vi "UHR-Fleezers Control (host) -Leonardo 04-2018 V1.vi"(0 "Tab Control":T5(tab)=enum."Trap Control (RF)") -> ()   [LabVIEW 2013] (continued)
                }
              }
            }
          }
          frame Enabled {
            n953 = call "hamilton_controller.vi"("Open?"=w1533, "valve"=enum16{"A", "B", "C", "D", "ALL"}."A", "action"=T21."MOVE VALVE") -> ()  [unwired: 8 in, 1 out]
          }
        }
      }
      event "Inject Valve B": Value Change {
        n954 = event-data() -> ()  [unwired: 7 out]
        n955 = disable-structure shown="Enabled" {
          disable-tunnel: "Inject Valve B" -> [w1537 w1557]
          frame Disabled {
            n956 = local read "Pump write delay (ms)"() -> (w1539:dbl)
            n957 = flat-sequence {
              tunnel: w1538 -> [w1552]
              tunnel: w1539 -> [w1548]
              tunnel: w1537 -> [_]
              tunnel: w1539 -> [w1554]
              tunnel: w1538 -> [w1555]
              frame #0 {
                n958 = local read "All Pump Parameters"() -> (w1547:T6)
                n959 = Multiply(x=60.0, y="Flush Center Ch Rate (ul/m)") -> (x*y=w1544:dbl)
                n960 = Unbundle By Name(w1547) -> ("Pump 2"=w1553:T33)
                n961 = call "Set pump parameters.vi"("Pump write delay (ms)"=w1548, "Volume (uL)"="Flush Center Ch Volume (uL)", "Rate (uL/h)"=w1544, "Units"=3.0, "Pump #"=2.0, "Pump Parameters In"=w1553, "VISA resource name"=w1552) -> ("Pump Parameters Out"=w1546:T33)  [unwired: 3 in]
                n962 = Bundle By Name(cluster=w1547, "Pump 2"=w1546) -> (w1545:T6)
                n963 = local write "All Pump Parameters"(w1545) -> ()
                n964 = Add(x="Flush Center Ch Volume (uL)", y="Total Volume\nFlushed (uL)") -> (x+y=w1541:dbl)
                n965 = local write "Total Volume\nFlushed (uL)"(w1541) -> ()
              }
              frame #1 {
                n966 = Wait (ms)(milliseconds to wait=w1554) -> ()  [unwired: 1 out]
              }
              frame #2 {
                n967 = call "Write to pump.vi"("string"="start", "VISA resource name"=w1555) -> ()  [unwired: 1 out]
              }
            }
            n968 = local read "Chemyx Syringe Pump Serial Port"() -> (w1538:refnum<visa-resource-name>)
          }
          frame Enabled {
            n969 = call "hamilton_controller.vi"("Open?"=w1557, "valve"=enum16{"A", "B", "C", "D", "ALL"}."B", "action"=T21."MOVE VALVE") -> ()  [unwired: 8 in, 1 out]
          }
        }
      }
      event "Inject Bottom": Value Change {
        n970 = event-data() -> ()  [unwired: 7 out]
        n971 = call "hamilton_controller.vi"("Open?"="Inject Bottom", "valve"=enum16{"A", "B", "C", "D", "ALL"}."C", "action"=T21."MOVE VALVE") -> ()  [unwired: 8 in, 1 out]
      }
      event "Shunt:": Value Change {
        n972 = event-data() -> ()  [unwired: 7 out]
        n973 = call "hamilton_controller.vi"("Open?"="Shunt:", "valve"=enum16{"A", "B", "C", "D", "ALL"}."D", "action"=T21."MOVE VALVE") -> ()  [unwired: 8 in, 1 out]
      }
      event "Flip Green Filter": Value Change {
        n974 = event-data() -> ()  [unwired: 7 out]
        n975 = local write "Flip Green Filter"("Flip Green Filter") -> ()
        n976 = flat-sequence {
          tunnel: w1573 -> [w1578]
          tunnel: w1572 -> [w1577]
          tunnel: [w1575] -> w1570
          tunnel: [w1574] -> w1569
          tunnel: [w1580] -> w1568
          tunnel: w1570 -> [w1580]
          tunnel: [w1579] -> w1567
          tunnel: w1569 -> [w1579]
          tunnel: w1568 -> [w1584]
          tunnel: w1567 -> [w1583]
          tunnel: [w1582] -> w1571
          frame #0 {
            n977 = xnode "Read/Write Control"("FPGA VI Reference In"=w1578, "error in"=w1577, "Green Filter Flipper"=TRUE) -> ("FPGA VI Reference Out"=w1575:T20, "error out"=w1574:errorcluster)
          }
          frame #1 {
            n978 = Wait (ms)(milliseconds to wait=u32 100) -> ()  [unwired: 1 out]
          }
          frame #2 {
            n979 = xnode "Read/Write Control"("FPGA VI Reference In"=w1584, "error in"=w1583, "Green Filter Flipper"=FALSE) -> ("error out"=w1582:errorcluster)  [unwired: 1 out]
          }
        }
      }
      event "Pump 1 contents", "Pump 3 contents": Value Change {
        n980 = event-data() -> ()  [unwired: 7 out]
        n981 = local read "Pump 1 contents"() -> (→"Pump 1 cont disp":string)
        n982 = local read "Pump 3 contents"() -> (→"Pump 3 cont disp":string)
      }
      event "Reset Trap Pos. FB": Value Change {
        n983 = event-data() -> ()  [unwired: 7 out]
        n984 = xnode "Read/Write Control"("FPGA VI Reference In"=w1590, "error in"=w1589, "Trap Pos. FB Reset"="Reset Trap Pos. FB") -> ()  [unwired: 2 out]
      }
      event "Trap Pos. FB ON": Value Change {
        n985 = event-data() -> ()  [unwired: 7 out]
        n986 = xnode "Read/Write Control"("FPGA VI Reference In"=w1605, "error in"=w1604) -> ("FPGA VI Reference Out"=w1602:T20, "BD1 Frequency Out 1"=w1599:u64)  [unwired: 1 out]
        n987 = To Double Precision Float(number=w1599) -> (double precision float=w1598:dbl)
        n988 = Multiply(x=49125000.0, y=6.0) -> (x*y=w1597:dbl)
        n989 = Multiply(x=w1598, y=w1597) -> (x*y=w1595:dbl)
        n990 = Scale By Power Of 2(n=-48, x=w1595) -> (x*2^n=w1594:dbl)
        n991 = Divide(x=w1594, y=1000000.0) -> (x/y=w1591:dbl)
        n992 = flat-sequence {
          tunnel: [w1608] -> w1603
          tunnel: w1602 -> [w1609]
          tunnel: w1599 -> [w1607]
          tunnel: "Trap Pos. FB ON" -> [w1606]
          tunnel: "Trap Pos. FB ON" -> [w1615]
          tunnel: w1603 -> [w1614]
          tunnel: "Trap Pos. FB ON" -> [w1617]
          tunnel: w1591 -> [w1616]
          frame #0 {
            n993 = case shown="False" w1606 {
              tunnel: w1609 -> [w1612 w1613]
              tunnel: [w1611 w1613] -> w1608
              tunnel: w1607 -> [w1610 _]
              frame False {
                n994 = xnode "Read/Write Control"("FPGA VI Reference In"=w1612, "BD 1 Frequency 1"=w1610) -> ("FPGA VI Reference Out"=w1611:T20)  [unwired: 1 in, 1 out]
              }
              frame True {
              }
            }
          }
          frame #1 {
            n995 = xnode "Read/Write Control"("FPGA VI Reference In"=w1614, "Force feedback"=w1615) -> ()  [unwired: 1 in, 2 out]
          }
          frame #2 {
            n996 = case shown="False" w1617 {
              tunnel: w1616 -> [w1620 _]
              frame False {
                n997 = local read "T2 for asymmetric\n(MHz)"() -> (w1618:dbl)
                n998 = Subtract(x=w1618, y=w1620) -> (x-y=w1619:dbl)
                n999 = property on="Trap Delta (MHz)" class="DigNum (strict)"("Val(Sgnl)"=w1619) -> ()  [unwired: 2 in, 2 out]
              }
              frame True {
              }
            }
          }
        }
      }
      event "Diff. FB.", "Trap Pos. FB Gains", "Trap Pos. FB Mult Factor", "Trap Pos. FB Offset Factor", "Trap Pos FB Negate Action", "Trap Pos FB Monitor\nT1 or T2", "Negate Diff?": Value Change {
        n1000 = event-data() -> ()  [unwired: 7 out]
        n1001 = xnode "Read/Write Control"("FPGA VI Reference In"=w1631, "error in"=w1630, "Trap pos. FB Range"="Trap Pos. FB Range", "Trap Pos. FB Gains"="Trap Pos. FB Gains", "Trap Pos. FB Mult Factor"="Trap Pos. FB Mult Factor", "Trap Pos. FB Offset Factor"="Trap Pos. FB Offset Factor", "Trap Pos FB Negate Action"="Trap Pos FB Negate Action", "Trap Pos FB Monitor T1 or T2"="Trap Pos FB Monitor\nT1 or T2", "AI1 X Scale"="Trap Pos. AI1 X Pre-scale", "Negate Diff?"="Negate Diff?", "Diff FB Measurement?"="Diff. FB.") -> ()  [unwired: 2 out]
      }
      event "Trap Pos FB SP": Value Change {
        n1002 = event-data() -> ()  [unwired: 7 out]
        n1003 = xnode "Read/Write Control"("FPGA VI Reference In"=w1634, "error in"=w1633, "Trap Pos. FB SP"="Trap Pos FB SP") -> ()  [unwired: 2 out]
        n1004 = disable-structure shown="Disabled" {
          frame Disabled {
            n1005 = local read "Trap X AI1 (DMA)"() -> (w1655:T13)
            n1006 = local read "Trap X (AI1)"() -> (w1656:T1)
            n1007 = local read "Setpoint offset\nCorrection values"() -> (w1649:dbl[])
            n1008 = local read "Trap Delta (MHz)"() -> (w1653:dbl)
            n1009 = local read "B factor"() -> (w1640:dbl)
            n1010 = Unbundle(w1656) -> ("Trap 1"=w1654:fxp<+/-,16,1>, "Trap 2"=w1643:fxp<+/-,16,1>)
            n1011 = Unbundle(w1655) -> ("Set 1"=w1639:fxp<+/-,16,1>, "Set 2"=w1638:fxp<+/-,16,1>)
            n1012 = Negate(x=w1643) -> (-x=w1636:fxp<+/-,17,2>)
            n1013 = Negate(x=w1654) -> (-x=w1637:fxp<+/-,17,2>)
            n1014 = Divide(x=w1653, y=0.1) -> (x/y=w1651:dbl)
            n1015 = Multiply(x=w1638, y=w1640) -> (x*y=w1641:dbl)
            n1016 = Subtract(x=w1639, y=w1641) -> (x-y=w1646:dbl)
            n1017 = To Long Integer(number=w1651) -> (32bit integer=w1650:i32)
            n1018 = Index Array(array=w1649, index=w1650) -> (element=w1645:dbl)
            n1019 = Multiply(x=w1640, y=w1636) -> (x*y=w1642:dbl)
            n1020 = Subtract(x=w1637, y=w1642) -> (x-y=w1648:dbl)
            n1021 = Add(x=w1648, y=w1645) -> (x+y=→"ideal setpoint fpga":dbl)
            n1022 = Add(x=w1646, y=w1645) -> (x+y=→"ideal setpoint avgd":dbl)
          }
          frame Enabled {
          }
        }
        n1023 = disable-structure shown="Enabled" {
          frame Enabled {
          }
          frame Disabled {
            n1024 = local write "B factor"(1.0 ("B factor")) -> ()
          }
        }
      }
      event "Simulate stepping": Value Change {
        n1025 = event-data() -> ()  [unwired: 7 out]
        n1026 = flat-sequence {
          tunnel: w1658 -> [w1661]
          tunnel: [w1660] -> _
          tunnel: w1657 -> [w1659]
          frame #0 {
            n1027 = while {
              tunnel: w1661 -> [w1689]
              tunnel: [w1688] -> w1660 mode=indexing
              tunnel: w1659 -> [w1687]
              i -> [w1673]
              stop <- w1670 stop-if-true
              w1663 = 1000.0
              n1028 = Divide(x="Backtrack probability", y=100) -> (x/y=w1697:dbl)
              n1029 = Random Number (0-1)() -> (number: 0 to 1=w1698:dbl)
              n1030 = Greater?(x=w1698, y=w1697) -> (0:w1696:bool)
              n1031 = Select(t=1, s=w1696, f=-1) -> (s? t:f=w1693:i32)
              n1032 = local read "BD 1 Frequency 2 (MHz)"() -> (w1668:dbl)
              n1033 = Multiply(x=w1693, y="Step size (nm)") -> (x*y=w1691:dbl)
              "Step taken" <- w1691
              n1034 = Divide(x=w1691, y=168.33) -> (x/y=w1666:dbl)
              n1035 = local read "BD 1 Frequency 1 (MHz)"() -> (w1667:dbl)
              n1036 = local read "X RF Frequency Limits (MHz)"() -> (w1686:T16)
              n1037 = local read "Y RF Frequency Limits (MHz)"() -> (w1685:T16)
              n1038 = Subtract(x=w1667, y=w1666) -> (x-y=w1665:dbl)
              n1039 = local write "BD 1 Frequency 1 (MHz)"(w1665) -> ()
              n1040 = local read "BD 2 Frequency 1 (MHz)"() -> (w1683:dbl)
              n1041 = local read "BD 2 Frequency 2 (MHz)"() -> (w1684:dbl)
              n1042 = call "set RF board frequency - interlace.vi"("Board 2 Frequency Limits"=w1685, "Board 1 Frequency Limits"=w1686, "error in"=w1689, "FPGA VI Reference In"=w1687, "Board 2 Frequency 2 (MHz)"=w1684, "Board 2 Frequency 1 (MHz)"=w1683, "Board 1 Frequency 2 (MHz)"=w1668, "Board 1 Frequency 1  (MHz)"=w1665) -> ("error out"=w1688:errorcluster)  [unwired: 2 in, 1 out]
              n1043 = Subtract(x=w1668, y=w1665) -> (x-y=w1682:dbl)
              n1044 = Subtract(x=w1684, y=w1683) -> (x-y=w1681:dbl)
              n1045 = Square(x=w1681) -> (x^2=w1679:dbl)
              n1046 = Square(x=w1682) -> (x^2=w1680:dbl)
              n1047 = Add(x=w1680, y=w1679) -> (x+y=w1678:dbl)
              n1048 = Square Root(x=w1678) -> (sqrt(x)=w1669:dbl)
              n1049 = local write "Trap Delta (MHz)"(w1669) -> ()
              n1050 = property on="Initial delta (MHz)" class="DigNum (strict)"("Val(Sgnl)"=w1669) -> ()  [unwired: 2 in, 2 out]
              n1051 = Multiply(x="Mean dwell time (s)", y=w1663) -> (x*y=w1675:dbl)
              n1052 = case shown="\"Gamma2\"" "Distribution" {
                tunnel: w1675 -> [w1702 w1706 w1709]
                tunnel: [w1702 w1703 w1710] -> w1664
                frame "uniform", Default {
                }
                frame "Exponential" {
                  n1053 = call-poly <vilib>:"Continuous Random.vi"("b"=w1706, "samples"=1) -> ("exp random data"=w1704:dbl[])  [unwired: 8 in, 1 out]
                  n1054 = Index Array(array=w1704) -> (element=w1703:dbl)  [unwired: 1 in]
                }
                frame "Gamma2" {
                  w1707 = 2.0
                  # "Note: the shape and scale\nparameters of the gamma\nare inverted because LabView..."
                  n1055 = Divide(x=w1709, y=w1707) -> (x/y=w1708:dbl)
                  n1056 = call-poly <vilib>:"Continuous Random.vi"("c"=w1708, "b"=w1707, "samples"=1) -> ("gamma random numbers"=w1711:dbl[])  [unwired: 7 in, 1 out]
                  n1057 = Index Array(array=w1711) -> (element=w1710:dbl)  [unwired: 1 in]
                }
              }
              n1058 = Divide(x=w1664, y=w1663) -> (x/y=→"Step duration":dbl)
              n1059 = To Unsigned Long Integer(number=w1664) -> (unsigned 32bit integer=w1676:u32)
              n1060 = Add(x=w1673, y=1) -> (x+y=w1672:i32)
              n1061 = Wait (ms)(milliseconds to wait=w1676) -> ()  [unwired: 1 out]
              n1062 = Equal?(x=w1672, y="Number of steps") -> (x = y?=w1670:bool)
            }
          }
          frame #1 {
            n1063 = local write "Simulate stepping"(FALSE) -> ()
          }
        }
      }
      event "Set SP to Reading": Value Change {
        n1064 = event-data() -> ()  [unwired: 7 out]
        n1065 = local read "Trap Pos FB Monitor\nT1 or T2"() -> (w1721:bool)
        n1066 = local read "Trap X AI1 (DMA)"() -> (w1724:T13)
        n1067 = local read "Trap X (AI1)"() -> (w1727:T1)
        n1068 = Unbundle By Name(w1727) -> ("Trap 1"=w1726:fxp<+/-,16,1>, "Trap 2"=w1725:fxp<+/-,16,1>)
        n1069 = Unbundle By Name(w1724) -> ("Set 1"=w1723:fxp<+/-,16,1>, "Set 2"=w1722:fxp<+/-,16,1>)
        n1070 = Select(t=w1726, s=w1721, f=w1725) -> (s? t:f=w1720:fxp<+/-,16,1>)
        n1071 = Select(t=w1723, s=w1721, f=w1722) -> (s? t:f=w1719:fxp<+/-,16,1>)
        n1072 = Not(x="Set SP Using...") -> (.not. x?=w1714:bool)
        n1073 = Select(t=w1720, s=w1714, f=w1719) -> (s? t:f=w1715:fxp<+/-,16,1>)
        n1074 = xnode "Read/Write Control"("FPGA VI Reference In"=w1717, "error in"=w1716, "Trap Pos. FB SP"=w1715) -> ()  [unwired: 2 out]
        n1075 = local write "Trap Pos FB SP"(w1715) -> ()
      }
      event "Trap Pos. FB Out Scale 2^n": Value Change {
        n1076 = event-data() -> ()  [unwired: 7 out]
        n1077 = Scale By Power Of 2(n="Trap Pos. FB Out Scale 2^n", x=ext 1.0) -> (x*2^n=w1729:ext)
        n1078 = property on="Trap Pos. FB Mult Factor" class="DigNum (strict)"("Val(Sgnl)"=w1729) -> ()  [unwired: 2 in, 2 out]
      }
      event "Trap Pos FB Int Count": Value Change {
        n1079 = event-data() -> ()  [unwired: 7 out]
        n1080 = xnode "Read/Write Control"("FPGA VI Reference In"=w1734, "error in"=w1733, "Trap Pos FB Int Count"="Trap Pos FB Int Count") -> ()  [unwired: 2 out]
      }
      event "Target Force (pN)", "Setpoint offset\nCorrection values", "Raster target force (pN)": Value Change {
        w1743 = 2.0
        n1081 = event-data() -> ()  [unwired: 7 out]
        n1082 = disable-structure "Removed B Factor to improve position feedback - Alex 081418 1of3" shown="Enabled" {
          disable-tunnel: [w1773 fxp<+/-,32,16> 1.0 ("B factor")] -> w1735
          frame Disabled {
            n1083 = local read "B factor"() -> (w1774:dbl)
            n1084 = To Fixed-Point(number=w1774) -> (fixed-point=w1773:fxp<+/-,16,16>)  [unwired: 1 in]
          }
          frame Enabled {
          }
        }
        n1085 = xnode "Read/Write Control"("FPGA VI Reference In"=w1737, "B factor"=w1735) -> ("BD1 Frequency Out 1"=w1764:u64)  [unwired: 1 in, 2 out]
        n1086 = local read "BD 1 Frequency 2 (MHz)"() -> (w1763:dbl)
        n1087 = local read "Target Force (pN)"() -> (w1749:dbl)
        n1088 = To Double Precision Float(number=w1764) -> (double precision float=w1770:dbl)
        n1089 = Multiply(x=49125000.0, y=6.0) -> (x*y=w1769:dbl)
        n1090 = Multiply(x=w1770, y=w1769) -> (x*y=w1767:dbl)
        n1091 = Scale By Power Of 2(n=-48, x=w1767) -> (x*2^n=w1766:dbl)
        n1092 = Divide(x=w1766, y=1000000.0) -> (x/y=w1762:dbl)
        n1093 = Subtract(x=w1763, y=w1762) -> (x-y=w1761:dbl)
        n1094 = local read "T1 kappa_x (pN/nm)"() -> (w1750:dbl)
        n1095 = local read "T1 alpha_x (nm/V)"() -> (w1751:dbl)
        n1096 = local read "Negate offset difference"() -> (w1752:bool)
        n1097 = local read "Offset file step size"() -> (w1760:dbl)
        n1098 = Multiply(x="Raster target force (pN)", y=w1743) -> (x*y=w1742:dbl)
        n1099 = Multiply(x=w1749, y=w1743) -> (x*y=w1748:dbl)
        n1100 = local read "Setpoint offset\nCorrection values"() -> (w1757:dbl[])
        n1101 = Divide(x=w1761, y=w1760) -> (x/y=w1759:dbl)
        n1102 = Select(t=-1, s=w1752, f=1) -> (s? t:f=w1753:i32)
        n1103 = To Long Integer(number=w1759) -> (32bit integer=w1758:i32)
        n1104 = Multiply(x=w1751, y=w1750) -> (x*y=w1741:dbl)
        n1105 = Divide(x=w1748, y=w1741) -> (x/y=w1747:dbl)
        n1106 = Index Array(array=w1757, index=w1758) -> (element=w1756:dbl)
        n1107 = Divide(x=w1742, y=w1741) -> (x/y=w1740:dbl)
        n1108 = Multiply(x=w1753, y=w1756) -> (x*y=w1739:dbl)
        n1109 = Add(x=w1747, y=w1739) -> (x+y=w1746:dbl)
        n1110 = Add(x=w1740, y=w1739) -> (x+y=w1738:dbl)
        n1111 = To Fixed-Point(number=w1738) -> (fixed-point=w1736:fxp<+/-,16,1>)  [unwired: 1 in]
        n1112 = To Fixed-Point(number=w1746) -> (fixed-point=w1745:fxp<+/-,16,1>)  [unwired: 1 in]
        n1113 = property on="Trap Pos FB SP" class="DigNum (strict)"("Val(Sgnl)"=w1745) -> ()  [unwired: 2 in, 2 out]
        n1114 = xnode "Read/Write Control"("FPGA VI Reference In"=w1737, "Raster setpoint"=w1736) -> ()  [unwired: 1 in, 2 out]
      }
      event "Read setpoint correction\nfile": Value Change {
        n1115 = event-data() -> ()  [unwired: 7 out]
        n1116 = local write "Read setpoint correction\nfile"(FALSE) -> ()
        n1117 = Open/Create/Replace File(file path (use dialog)="Setpoint correction\noffset file", operation (0:open)=T24."open", access (0:read/write)=enum16{"read/write", "read-only", "write-only"}."read-only") -> (refnum out=w1801:refnum<file>)  [unwired: 1 in, 4 out]
        n1118 = Deny Access(7:w1801) -> (3:w1799:refnum<file>)  [unwired: 1 in, 2 out]
        n1119 = Read from Binary File(5:0.0, 9:T30."big-endian, network order" ("byte order (0:big-endian, network order)"), 10:-1 ("count (1)"), 11:w1799) -> (2:w1792:dbl[], 3:w1798:refnum<file>)  [unwired: 1 in, 3 out]
        n1120 = Close File(refnum=w1798) -> ()  [unwired: 1 in, 2 out]
        n1121 = Index Array(array=w1792, index=0) -> (element=w1788:dbl)
        n1122 = local write "Offset file step size"(w1788) -> ()
        n1123 = Array Subset(array=w1792, index=3) -> (w1791:dbl[])  [unwired: 1 in]
        n1124 = local read "T1 kappa_x (pN/nm)"() -> (w1786:dbl)
        n1125 = local read "T1 alpha_x (nm/V)"() -> (w1787:dbl)
        n1126 = local read "T2 alpha_x (nm/V)"() -> (w1785:dbl)
        n1127 = local read "T2 kappa_x (pN/nm)"() -> (w1784:dbl)
        n1128 = Decimate 1D Array(w1791) -> (w1780:dbl[], w1781:dbl[])  [unwired: 1 out]
        n1129 = local read "Offset Values"() -> (w1790:T14)
        n1130 = Multiply(x=w1787, y=w1786) -> (x*y=w1782:dbl)
        n1131 = Multiply(x=w1785, y=w1784) -> (x*y=w1783:dbl)
        n1132 = Bundle By Name(cluster=w1790, "Trap 1X offset"=w1780, "Trap 2X offset"=w1781) -> (w1789:T14)
        n1133 = Divide(x=w1783, y=w1782) -> (x/y=w1777:dbl)
        n1134 = disable-structure "Removed B Factor to better position FB - Alex 081418 3of3" shown="Enabled" {
          disable-tunnel: w1777 -> [w1805 _]
          disable-tunnel: [w1805 1.0] -> w1776
          frame Disabled {
          }
          frame Enabled {
          }
        }
        n1135 = Multiply(x=w1781, y=w1776) -> (x*y=w1779:dbl[])
        n1136 = local write "Offset Values"(w1789) -> ()
        n1137 = Subtract(x=w1780, y=w1779) -> (x-y=w1778:dbl[])
        n1138 = property on="B factor" class="DigNum (strict)"("Val(Sgnl)"=w1776) -> ()  [unwired: 2 in, 2 out]
        n1139 = property on="Setpoint offset\nCorrection values" class="Arr (strict)"("Val(Sgnl)"=w1778) -> ()  [unwired: 2 in, 2 out]
      }
      event "MCL Tracking": Value Change {
        n1140 = event-data() -> ()  [unwired: 7 out]
        n1141 = case shown="True" "MCL Tracking" {
          frame False {
            n1142 = local read "Current MCL (V)"() -> (w1808:dbl)
            n1143 = local write "AO2"(w1808) -> ()
          }
          frame True {
            n1144 = local read "BD 1 Frequency 1 (MHz)"() -> (→"Zero T1 position":dbl)
            n1145 = local read "AO2"() -> (→"Zero MCL x position":dbl)
          }
        }
      }
      event "Scale intensities": Value Change {
        n1146 = event-data() -> ()  [unwired: 7 out]
        n1147 = local read "Trap Intensity\nSetpoints (V)"() -> (w1814:cluster{"Set 1":dbl, "Set 2":dbl})
        n1148 = local read "T1 kappa_x (pN/nm)"() -> (w1820:dbl)
        n1149 = local read "T2 kappa_x (pN/nm)"() -> (w1819:dbl)
        n1150 = Unbundle By Name(w1814) -> ("Set 1"=w1816:dbl, "Set 2"=w1815:dbl)
        n1151 = case shown="True" "Scale intensities" {
          tunnel: "Scale factor" -> [w1830 w1842]
          tunnel: "Scale factor" -> [w1825 w1835]
          tunnel: w1820 -> [w1832 w1841]
          tunnel: w1819 -> [w1831 w1840]
          tunnel: [w1828 w1839] -> w1818
          tunnel: [w1829 w1838] -> w1817
          tunnel: w1816 -> [w1827 w1837]
          tunnel: w1815 -> [w1826 w1836]
          tunnel: [w1824 w1834] -> w1813
          tunnel: [w1823 w1833] -> w1812
          frame False {
            n1152 = Divide(x=w1832, y=w1825) -> (x/y=w1828:dbl)
            n1153 = Divide(x=w1831, y=w1830) -> (x/y=w1829:dbl)
            n1154 = Divide(x=w1827, y=w1825) -> (x/y=w1824:dbl)
            n1155 = Divide(x=w1826, y=w1825) -> (x/y=w1823:dbl)
          }
          frame True {
            n1156 = Multiply(x=w1837, y=w1835) -> (x*y=w1834:dbl)
            n1157 = Multiply(x=w1836, y=w1835) -> (x*y=w1833:dbl)
            n1158 = Multiply(x=w1841, y=w1835) -> (x*y=w1839:dbl)
            n1159 = Multiply(x=w1842, y=w1840) -> (x*y=w1838:dbl)
          }
        }
        n1160 = local write "T2 kappa_x (pN/nm)"(w1817) -> ()
        n1161 = local write "T1 kappa_x (pN/nm)"(w1818) -> ()
        n1162 = Bundle By Name(cluster=w1814, "Set 1"=w1813, "Set 2"=w1812) -> (w1811:cluster{"Set 1":dbl, "Set 2":dbl})
        n1163 = property on="Trap Intensity\nSetpoints (V)" class="Clust (strict)"("Val(Sgnl)"=w1811) -> ()  [unwired: 2 in, 2 out]
      }
    }
    "error out 2" <- w771
    n1164 = node-c288() -> ()  [unwired: 1 in, 1 out]
  }
  n1165 = node-c288() -> (w102:T25)  [unwired: 4 in]
  n1166 = timed-loop "Run Scripts, including: stage motion" {
    timing: w102 -> [_]
    timing-out: [_] -> w101
    tunnel: w59 -> [_]
    stop <- w1844 stop-if-true
    n1167 = node-c288() -> ()  [unwired: 1 in, 1 out]
    n1168 = event shown="[2] \"Cal/Data Acq. Spot\": Value Change" {
      selector: _ -> [_ _ _ _ _ _ _ _ _ _ _ _]
      dyn-events: _ -> [_ _ _ _ _ _ _ _ _ _ _ _]
      timeout: 50 -> [_ _ _ _ _ _ _ _ _ _ _ _]
      tunnel: ["Move Cap. 1 (DNA Top)" _ "Cal/Data Acq. Spot" "Dump Beads" "Dip for Protein" _ "Got ADig bead" "Got DNA bead" "Take Stepping Data" _ "Take Detection Laser\nImage" _] -> _
      tunnel: [_ _ _ _ _ _ _ _ _ _ _ w2054] -> w1844
      event "Move Cap. 1 (DNA Top)": Value Change {
        n1169 = event-data() -> ()  [unwired: 1 in, 5 out]
        n1170 = local write "Move Cap. 1 (DNA Top)"(FALSE ("Move Cap. 1 (DNA Right)")) -> ()
        n1171 = flat-sequence {
          tunnel: "Cap 1 Samp Flow ON" -> [w1850]
          frame #0 {
            n1172 = local write "Stage Moving"(FALSE ("Stage Moving")) -> ()
            n1173 = case "stop flow" shown="True" w1850 {
              frame False {
              }
              frame True {
                n1174 = call "hamilton_controller.vi"("Open?"=FALSE, "valve"=enum16{"A", "B", "C", "D", "ALL"}."C", "action"=T21."MOVE VALVE") -> ()  [unwired: 8 in, 1 out]
              }
            }
            n1175 = case shown="True" TRUE {
              tunnel: "Cap 1 T ON" -> [w1859 w1860]
              frame False {
                n1176 = property on="Trap 1 (ON/OFF)" class="Bool (strict)"("Val(Sgnl)"=w1859) -> ()  [unwired: 2 in, 2 out]
              }
              frame True {
                n1177 = property on="Trap 2 (ON/OFF)" class="Bool (strict)"("Val(Sgnl)"=w1860) -> ()  [unwired: 2 in, 2 out]
              }
            }
            n1178 = call <vilib>:"Beep.vi"() -> ()  [unwired: 3 in, 9 out]
            n1179 = case shown="True" "Cap 1 Flow ON" {
              frame False {
              }
              frame True {
                n1180 = property on="Main:" class="Bool (strict)"("Val(Sgnl)"=TRUE ("Value (Signaling)")) -> ()  [unwired: 2 in, 2 out]
              }
            }
          }
        }
      }
      event Timeout {
        n1181 = event-data() -> ()  [unwired: 1 in, 2 out]
      }
      event "Cal/Data Acq. Spot": Value Change {
        # "wait for calibration file\nto be written"
        # "signal save cal true\nthis tells the data \nacquisition loop to\nstart sending the data\nto a calibration file"
        # "separate traps to\nthe desired trap delta"
        # "move stage to data acquisition spot"
        # "CHANGE FISH FOR TETHER BACK\nTO TRUE VALUE HERE."
        n1182 = event-data() -> ()  [unwired: 1 in, 5 out]
        n1183 = flat-sequence {
          tunnel: ["Cal @ (MHz)"] -> w1861
          tunnel: w1861 -> [w1873]
          tunnel: w1861 -> [w1894]
          frame #0 {
            n1184 = property on="Trap Delta (MHz)" class="DigNum (strict)"("Val(Sgnl)"="Cal @ (MHz)") -> ()  [unwired: 2 in, 2 out]
            n1185 = call <vilib>:"Beep.vi"() -> ()  [unwired: 3 in, 9 out]
          }
          frame #1 {
            n1186 = local read "Scale intensities"() -> (w1865:bool)
            n1187 = case shown="True" w1865 {
              frame False {
              }
              frame True {
                n1188 = property on="Scale intensities" class="Bool (strict)"("Val(Sgnl)"=FALSE ("Value (Signaling)")) -> ()  [unwired: 2 in, 2 out]
              }
            }
            n1189 = Wait (ms)(milliseconds to wait=u32 250) -> ()  [unwired: 1 out]
          }
          frame #2 {
            n1190 = property on="Save Calibration" class="Bool (strict)"("Val(Sgnl)"=TRUE ("Value (Signaling)")) -> ()  [unwired: 2 in, 2 out]
          }
          frame #3 {
            n1191 = Wait (ms)(milliseconds to wait=u32 4000) -> ()  [unwired: 1 out]
          }
          frame #4 {
            n1192 = while {
              stop <- w1870 stop-if-true
              n1193 = local read "Saving..."() -> (w1871:bool)
              n1194 = Wait (ms)(milliseconds to wait=u32 100) -> ()  [unwired: 1 out]
              n1195 = Not(x=w1871) -> (.not. x?=w1870:bool)
            }
          }
          frame #5 {
            n1196 = case shown="True" "W/ Offset 1" {
              tunnel: w1873 -> [_ w1875]
              frame False {
              }
              frame True {
                n1197 = stacked-sequence {
                  tunnel: w1875 -> [_ _ _ _ _ _ _ w1892]
                  frame #0 {
                    n1198 = Replace Array Subset(array=u32[] [0] ("Index Values"), new element="Offset 1 Set", index=0) -> (w1876:u32[])
                    n1199 = property on="Saved AOD Raster Scan Parameter Sets" class="Arr (strict)"("Index Values"=w1876) -> ()  [unwired: 2 in, 2 out]
                    n1200 = property on="Trap Delta (MHz)" class="DigNum (strict)"("Val(Sgnl)"="Offset 1 Start (MHz)") -> ()  [unwired: 2 in, 2 out]
                  }
                  frame #1 {
                    n1201 = Wait (ms)(milliseconds to wait=u32 200) -> ()  [unwired: 1 out]
                  }
                  frame #2 {
                    n1202 = property on="Load parameters" class="Bool (strict)"("Val(Sgnl)"=TRUE ("Value (Signaling)")) -> ()  [unwired: 2 in, 2 out]
                  }
                  frame #3 {
                    n1203 = Wait (ms)(milliseconds to wait=u32 200) -> ()  [unwired: 1 out]
                  }
                  frame #4 {
                    n1204 = property on="Trap Raster Scan" class="Bool (strict)"("Val(Sgnl)"=TRUE ("Value (Signaling)")) -> ()  [unwired: 2 in, 2 out]
                  }
                  frame #5 {
                    n1205 = Wait (ms)(milliseconds to wait=u32 2000) -> ()  [unwired: 1 out]
                  }
                  frame #6 {
                    n1206 = while {
                      stop <- w1889 stop-if-true
                      n1207 = local read "Raster Scanning..."() -> (w1891:bool)
                      n1208 = local read "Saving..."() -> (w1887:bool)
                      n1209 = Wait (ms)(milliseconds to wait=u32 100) -> ()  [unwired: 1 out]
                      n1210 = Not(x=w1887) -> (.not. x?=w1886:bool)
                      n1211 = Not(x=w1891) -> (.not. x?=w1888:bool)
                      n1212 = And(x=w1888, y=w1886) -> (x .and. y?=w1889:bool)
                    }
                  }
                  frame #7 {
                    n1213 = property on="Trap Delta (MHz)" class="DigNum (strict)"("Val(Sgnl)"=w1892) -> ()  [unwired: 2 in, 2 out]
                  }
                }
              }
            }
          }
          frame #6 {
            n1214 = local read "Save ave N"() -> (w1893:dbl)
            n1215 = case shown="True" "W/ Offset 2" {
              tunnel: w1894 -> [_ w1900]
              tunnel: w1893 -> [_ w1899]
              frame False {
                n1216 = Multiply(x="Cal read wait (s)", y=u32 1000 ("milliseconds to wait")) -> (x*y=w1897:u32)
                n1217 = Wait (ms)(milliseconds to wait=w1897) -> ()  [unwired: 1 out]
              }
              frame True {
                n1218 = stacked-sequence {
                  tunnel: w1900 -> [_ _ _ _ _ _ _ _ _ w1921 _ _]
                  tunnel: w1899 -> [_ _ _ _ _ _ _ _ _ w1919 _ _]
                  frame #0 {
                    n1219 = property on="Save ave N" class="DigNum (strict)"("Val(Sgnl)"=1.0 ("Value (Signaling)")) -> ()  [unwired: 2 in, 2 out]
                  }
                  frame #1 {
                    n1220 = Wait (ms)(milliseconds to wait=u32 500) -> ()  [unwired: 1 out]
                  }
                  frame #2 {
                    n1221 = property on="Trap Delta (MHz)" class="DigNum (strict)"("Val(Sgnl)"="Offset 2 Start (MHz)") -> ()  [unwired: 2 in, 2 out]
                    n1222 = Replace Array Subset(array=u32[] [0] ("Index Values"), new element="Offset 2 Set", index=0) -> (w1905:u32[])
                    n1223 = property on="Saved AOD Raster Scan Parameter Sets" class="Arr (strict)"("Index Values"=w1905) -> ()  [unwired: 2 in, 2 out]
                  }
                  frame #3 {
                    n1224 = Wait (ms)(milliseconds to wait=u32 500) -> ()  [unwired: 1 out]
                  }
                  frame #4 {
                    n1225 = property on="Load parameters" class="Bool (strict)"("Val(Sgnl)"=TRUE ("Value (Signaling)")) -> ()  [unwired: 2 in, 2 out]
                  }
                  frame #5 {
                    n1226 = Wait (ms)(milliseconds to wait=u32 500) -> ()  [unwired: 1 out]
                  }
                  frame #6 {
                    n1227 = property on="Trap Raster Scan" class="Bool (strict)"("Val(Sgnl)"=TRUE ("Value (Signaling)")) -> ()  [unwired: 2 in, 2 out]
                  }
                  frame #7 {
                    n1228 = Wait (ms)(milliseconds to wait=u32 2000) -> ()  [unwired: 1 out]
                  }
                  frame #8 {
                    n1229 = while {
                      stop <- w1914 stop-if-true
                      n1230 = local read "Raster Scanning..."() -> (w1917:bool)
                      n1231 = local read "Saving..."() -> (w1915:bool)
                      n1232 = Wait (ms)(milliseconds to wait=u32 100) -> ()  [unwired: 1 out]
                      n1233 = Not(x=w1915) -> (.not. x?=w1913:bool)
                      n1234 = Not(x=w1917) -> (.not. x?=w1916:bool)
                      n1235 = And(x=w1916, y=w1913) -> (x .and. y?=w1914:bool)
                    }
                  }
                  frame #9 {
                    n1236 = property on="Trap Delta (MHz)" class="DigNum (strict)"("Val(Sgnl)"=w1921) -> ()  [unwired: 2 in, 2 out]
                    n1237 = property on="Saved AOD Raster Scan Parameter Sets" class="Arr (strict)"("Index Values"=u32[] [0]) -> ()  [unwired: 2 in, 2 out]
                    n1238 = property on="Save ave N" class="DigNum (strict)"("Val(Sgnl)"=w1919) -> ()  [unwired: 2 in, 2 out]
                  }
                  frame #10 {
                    n1239 = Wait (ms)(milliseconds to wait=u32 500) -> ()  [unwired: 1 out]
                  }
                  frame #11 {
                    n1240 = property on="Load parameters" class="Bool (strict)"("Val(Sgnl)"=TRUE ("Value (Signaling)")) -> ()  [unwired: 2 in, 2 out]
                  }
                }
              }
            }
          }
          frame #7 {
            n1241 = property on="Read Cal" class="Bool (strict)"("Val(Sgnl)"=TRUE ("Value (Signaling)")) -> ()  [unwired: 2 in, 2 out]
          }
          frame #8 {
            n1242 = Wait (ms)(milliseconds to wait=u32 500) -> ()  [unwired: 1 out]
          }
          frame #9 {
            n1243 = property on="Fish for Tether" class="Bool (strict)"("Val(Sgnl)"=FALSE ("Value (Signaling)")) -> ()  [unwired: 2 in, 2 out]
          }
        }
        n1244 = local write "Cal/Data Acq. Spot"(FALSE ("Cal/Data Acq. Spot")) -> ()
      }
      event "Dump Beads": Value Change {
        # "SCRIPT TO REMOVE BOTH BEADS FROM THE TRAPS. TURNS ON LIGHT WHICH INDICATES THAT STAGE IS MOVING. THEN STOPS SAVING DATA. \nSETS Sample Channel Flow TO TRUE. STOPS INTERLACING GREEN FLUORESCENCE. TURNS OFF Tether INDICATOR BECAUSE WE ARE THROWING IT\nAWAY. SHUTS OFF TRAP POSITION FEEDBACK."
        n1245 = event-data() -> ()  [unwired: 1 in, 5 out]
        n1246 = flat-sequence {
          frame #0 {
            w1928 = FALSE ("Fl. Triggered...")
            w1929 = TRUE ("Stage Moving")
            n1247 = local read "Saving..."() -> (w1930:bool)
            n1248 = local write "Fl. Triggered..."(w1928) -> ()
            n1249 = local write "Stage Moving"(w1929) -> ()
            n1250 = local write "Tether"(w1928) -> ()
            n1251 = property on="Green Laser ON/Interlacing" class="Bool (strict)"("Val(Sgnl)"=w1928) -> ()  [unwired: 2 in, 2 out]
            n1252 = property on="Trap Pos. FB ON" class="Bool (strict)"("Val(Sgnl)"=w1928) -> ()  [unwired: 2 in, 2 out]
            n1253 = property on="Inject Bottom" class="Bool (strict)"("Val(Sgnl)"=w1929) -> ()  [unwired: 2 in, 2 out]
            n1254 = local write "Stop Saving"(w1930) -> ()
          }
          frame #1 {
            w1931 = FALSE ("Value (Signaling)")
            # "TURNS TRAPS OFF SO THAT\nBEADS REMAIN AT DUMP \nBEADS POSITION"
            n1255 = property on="Trap 1 (ON/OFF)" class="Bool (strict)"("Val(Sgnl)"=w1931) -> ()  [unwired: 2 in, 2 out]
            n1256 = property on="Trap 2 (ON/OFF)" class="Bool (strict)"("Val(Sgnl)"=w1931) -> ()  [unwired: 2 in, 2 out]
            n1257 = call <vilib>:"Beep.vi"() -> ()  [unwired: 3 in, 9 out]
          }
          frame #2 {
            n1258 = property on="Goto Bottom (F7)" class="Bool (strict)"("Val(Sgnl)"=TRUE ("Value (Signaling)")) -> ()  [unwired: 2 in, 2 out]
          }
          frame #3 {
            n1259 = Wait (ms)(milliseconds to wait=u32 8000) -> ()  [unwired: 1 out]
          }
          frame #4 {
            n1260 = property on="Trap Delta (MHz)" class="DigNum (strict)"("Val(Sgnl)"=20.0 ("Value (Signaling)")) -> ()  [unwired: 2 in, 2 out]
          }
          frame #5 {
            n1261 = property on="Trap 2 (ON/OFF)" class="Bool (strict)"("Val(Sgnl)"=TRUE ("Value (Signaling)")) -> ()  [unwired: 2 in, 2 out]
          }
          frame #6 {
            n1262 = property on="Inject Bottom" class="Bool (strict)"("Val(Sgnl)"=FALSE ("Value (Signaling)")) -> ()  [unwired: 2 in, 2 out]
          }
        }
      }
      event "Dip for Protein": Value Change {
        n1263 = event-data() -> ()  [unwired: 1 in, 5 out]
        n1264 = flat-sequence {
          frame #0 {
            n1265 = case shown="True" "Move Trap Before?" {
              frame False {
              }
              frame True {
                n1266 = property on="Trap Delta (MHz)" class="DigNum (strict)"("Val(Sgnl)"="Dip Trap Delta 1 (MHz)") -> ()  [unwired: 2 in, 2 out]
              }
            }
          }
          frame #1 {
            n1267 = Multiply(x="Duration (s)", y=1000.0) -> (x*y=w1940:dbl)
            n1268 = Wait (ms)(milliseconds to wait=w1940) -> ()  [unwired: 1 out]
          }
          frame #2 {
            n1269 = case shown="True" "Move Trap After?" {
              frame False {
              }
              frame True {
                n1270 = property on="Trap Delta (MHz)" class="DigNum (strict)"("Val(Sgnl)"="Dip Trap Delta 2 (MHz)") -> ()  [unwired: 2 in, 2 out]
              }
            }
          }
          frame #3 {
            n1271 = case shown="True" "Green ON After?" {
              frame False {
              }
              frame True {
                n1272 = property on="Green Laser ON/Interlacing" class="Bool (strict)"("Val(Sgnl)"=TRUE ("Value (Signaling)")) -> ()  [unwired: 2 in, 2 out]
              }
            }
          }
          frame #4 {
            n1273 = Wait (ms)(milliseconds to wait=u32 500) -> ()  [unwired: 1 out]
          }
          frame #5 {
            n1274 = case shown="True" "Save Data After?" {
              frame False {
              }
              frame True {
                n1275 = property on="Start Saving" class="Bool (strict)"("Val(Sgnl)"=TRUE ("Value (Signaling)")) -> ()  [unwired: 2 in, 2 out]
              }
            }
          }
        }
      }
      event "Profile": Value Change {
        n1276 = event-data() -> ()  [unwired: 1 in, 5 out]
        n1277 = flat-sequence {
          frame #0 {
            w1950 = 0.0 ("element")
            n1278 = Build Array(w1950, "Y change (mm)", w1950) -> ()  [unwired: 1 out]
          }
          frame #1 {
            # "stop saving"
            n1279 = local write "Stop Saving"(TRUE ("Stop Saving")) -> ()
            n1280 = local write "Stage Moving"(FALSE ("Stage Moving")) -> ()
          }
        }
      }
      event "Got ADig bead": Value Change {
        n1281 = event-data() -> ()  [unwired: 1 in, 5 out]
        n1282 = property on="Move Cap. 1 (DNA Top)" class="Bool (strict)"("Val(Sgnl)"=TRUE ("Value (Signaling)")) -> ()  [unwired: 2 in, 2 out]
        n1283 = property on="Inject Top:" class="Bool (strict)"("Val(Sgnl)"=FALSE ("Value (Signaling)")) -> ()  [unwired: 2 in, 2 out]
      }
      event "Got DNA bead": Value Change {
        n1284 = event-data() -> ()  [unwired: 1 in, 5 out]
        n1285 = property on="Cal/Data Acq. Spot" class="Bool (strict)"("Val(Sgnl)"=TRUE ("Value (Signaling)")) -> ()  [unwired: 2 in, 2 out]
        n1286 = property on="Main:" class="Bool (strict)"("Val(Sgnl)"=FALSE ("Value (Signaling)")) -> ()  [unwired: 2 in, 2 out]
      }
      event "Take Stepping Data": Value Change {
        n1287 = event-data() -> ()  [unwired: 1 in, 5 out]
        n1288 = local read "Save ave N"() -> (w1968:dbl)
        n1289 = flat-sequence {
          tunnel: w1968 -> [w1970]
          tunnel: [w1970] -> w1963
          tunnel: [w1972] -> w1964
          tunnel: w1963 -> [w1972]
          tunnel: [w1974] -> w1965
          tunnel: w1964 -> [w1974]
          tunnel: [w1977] -> w1966
          tunnel: w1965 -> [w1977]
          tunnel: [w1979] -> w1967
          tunnel: w1966 -> [w1979]
          tunnel: [w1981] -> w1961
          tunnel: w1967 -> [w1981]
          tunnel: w1961 -> [w1984]
          tunnel: [w1984] -> w1960
          tunnel: w1960 -> [w1985]
          tunnel: [w1985] -> w1962
          tunnel: w1962 -> [w1991]
          frame #0 {
            n1290 = property on="Save ave N" class="DigNum (strict)"("Val(Sgnl)"="Save ave factor") -> ()  [unwired: 2 in, 2 out]
          }
          frame #1 {
            n1291 = Wait (ms)(milliseconds to wait=u32 100) -> ()  [unwired: 1 out]
          }
          frame #2 {
            n1292 = local read "Offset 2 Start (MHz)"() -> (w1976:dbl)
            n1293 = property on="Saved AOD Raster Scan Parameter Sets" class="Arr (strict)"("Index Values"=u32[] [2]) -> ()  [unwired: 2 in, 2 out]
            n1294 = property on="Trap Delta (MHz)" class="DigNum (strict)"("Val(Sgnl)"=w1976) -> ()  [unwired: 2 in, 2 out]
          }
          frame #3 {
            n1295 = property on="Load parameters" class="Bool (strict)"("Val(Sgnl)"=TRUE ("Value (Signaling)")) -> ()  [unwired: 2 in, 2 out]
          }
          frame #4 {
            n1296 = Wait (ms)(milliseconds to wait=u32 100) -> ()  [unwired: 1 out]
          }
          frame #5 {
            n1297 = property on="Trap Raster Scan" class="Bool (strict)"("Val(Sgnl)"=TRUE ("Value (Signaling)")) -> ()  [unwired: 2 in, 2 out]
          }
          frame #6 {
            n1298 = Wait (ms)(milliseconds to wait=u32 1000) -> ()  [unwired: 1 out]
          }
          frame #7 {
            n1299 = while {
              stop <- w1988 stop-if-true
              n1300 = local read "Raster Scanning..."() -> (w1990:bool)
              n1301 = local read "Saving..."() -> (w1989:bool)
              n1302 = Not(x=w1989) -> (.not. x?=w1986:bool)
              n1303 = Not(x=w1990) -> (.not. x?=w1987:bool)
              n1304 = And(x=w1987, y=w1986) -> (x .and. y?=w1988:bool)
            }
          }
          frame #8 {
            n1305 = property on="Save ave N" class="DigNum (strict)"("Val(Sgnl)"=w1991) -> ()  [unwired: 2 in, 2 out]
          }
        }
      }
      event "Step Size (nm)": Value Change {
        n1306 = event-data() -> ()  [unwired: 1 in, 5 out]
        n1307 = flat-sequence {
          frame #0 {
            n1308 = property on="Saved AOD Raster Scan Parameter Sets" class="Arr (strict)"("Index Values"=u32[] [1]) -> ()  [unwired: 2 in, 2 out]
          }
          frame #1 {
            n1309 = Multiply(x="N Steps", y="Step Size (nm)") -> (x*y=w1993:dbl)
            n1310 = property on="Scan Speed AOD (nm/s) 2" class="DigNum (strict)"("Value"="Step Size (nm)") -> ()  [unwired: 2 in, 2 out]
            n1311 = property on="Step Size AOD (nm) 2" class="DigNum (strict)"("Value"="Step Size (nm)") -> ()  [unwired: 2 in, 2 out]
            n1312 = property on="Scan Range AOD (nm) 2" class="DigNum (strict)"("Value"=w1993) -> ()  [unwired: 2 in, 2 out]
          }
        }
      }
      event "Take Detection Laser\nImage": Value Change {
        n1313 = event-data() -> ()  [unwired: 1 in, 5 out]
        n1314 = flat-sequence {
          tunnel: [w2021] -> w2011
          tunnel: [w2020] -> w2004
          tunnel: [w2019] -> w1996
          tunnel: [w2024] -> w2012
          tunnel: w2011 -> [w2024]
          tunnel: [w2023] -> w2005
          tunnel: w2004 -> [w2023]
          tunnel: [w2022] -> w1997
          tunnel: w1996 -> [w2022]
          tunnel: [w2028] -> w2013
          tunnel: w2012 -> [w2028]
          tunnel: [w2027] -> w2006
          tunnel: w2005 -> [w2027]
          tunnel: [w2026] -> w1998
          tunnel: w1997 -> [w2026]
          tunnel: [w2034] -> w2014
          tunnel: w2013 -> [w2034]
          tunnel: [w2033] -> w2007
          tunnel: w2006 -> [w2033]
          tunnel: [w2032] -> w1999
          tunnel: w1998 -> [w2032]
          tunnel: [w2038] -> w2015
          tunnel: w2014 -> [w2038]
          tunnel: [w2037] -> w2008
          tunnel: w2007 -> [w2037]
          tunnel: [w2036] -> w2000
          tunnel: w1999 -> [w2036]
          tunnel: [w2042] -> w2016
          tunnel: w2015 -> [w2042]
          tunnel: [w2041] -> w2009
          tunnel: w2008 -> [w2041]
          tunnel: [w2040] -> w2001
          tunnel: w2000 -> [w2040]
          tunnel: [w2046] -> w2017
          tunnel: w2016 -> [w2046]
          tunnel: [w2045] -> w2010
          tunnel: w2009 -> [w2045]
          tunnel: [w2044] -> w2002
          tunnel: w2001 -> [w2044]
          tunnel: w2017 -> [w2052]
          tunnel: w2010 -> [w2051]
          tunnel: [w2049] -> w2003
          tunnel: w2002 -> [w2049]
          tunnel: w2003 -> [w2053]
          frame #0 {
            n1315 = local read "Green Laser ON/Interlacing"() -> (w2021:bool)
            n1316 = local read "Green laser mode"() -> (w2020:enum32{"Laser ON", "Laser OFF", "Interlace"})
            n1317 = local read "Green FB On/Off"() -> (w2019:bool)
          }
          frame #1 {
            n1318 = property on="Green FB On/Off" class="Bool (strict)"("Val(Sgnl)"=FALSE ("Value (Signaling)")) -> ()  [unwired: 2 in, 2 out]
          }
          frame #2 {
            n1319 = property on="Green Laser ON/Interlacing" class="Bool (strict)"("Val(Sgnl)"=TRUE ("Value (Signaling)")) -> ()  [unwired: 2 in, 2 out]
            n1320 = property on="Flip Green Filter" class="Bool (strict)"("Val(Sgnl)"=TRUE ("Value (Signaling)")) -> ()  [unwired: 2 in, 2 out]
            n1321 = property on="Green laser mode" class="RadioBtnsControl (strict)"("Val(Sgnl)"=enum32{"Laser ON", "Laser OFF", "Interlace"}."Laser ON" ("Value (Signaling)")) -> ()  [unwired: 2 in, 2 out]
          }
          frame #3 {
            n1322 = Wait (ms)(milliseconds to wait=u32 500) -> ()  [unwired: 1 out]
          }
          frame #4 {
            n1323 = property on="Confocal Image" class="Bool (strict)"("Val(Sgnl)"=TRUE ("Value (Signaling)")) -> ()  [unwired: 2 in, 2 out]
          }
          frame #5 {
            n1324 = Wait (ms)(milliseconds to wait=u32 2000) -> ()  [unwired: 1 out]
          }
          frame #6 {
            n1325 = while {
              stop <- w2047 stop-if-true
              n1326 = local read "Saving..."() -> (w2048:bool)
              n1327 = Not(x=w2048) -> (.not. x?=w2047:bool)
            }
          }
          frame #7 {
            n1328 = property on="Flip Green Filter" class="Bool (strict)"("Val(Sgnl)"=TRUE ("Value (Signaling)")) -> ()  [unwired: 2 in, 2 out]
            n1329 = property on="Green Laser ON/Interlacing" class="Bool (strict)"("Val(Sgnl)"=w2052) -> ()  [unwired: 2 in, 2 out]
            n1330 = property on="Green laser mode" class="RadioBtnsControl (strict)"("Val(Sgnl)"=w2051) -> ()  [unwired: 2 in, 2 out]
          }
          frame #8 {
            n1331 = property on="Green FB On/Off" class="Bool (strict)"("Val(Sgnl)"=w2053) -> ()  [unwired: 2 in, 2 out]
          }
        }
      }
      event "Stop All": Value Change {
        n1332 = event-data() -> ()  [unwired: 1 in, 5 out]
        n1333 = local read "Stop All"() -> (w2054:bool)
      }
    }
    n1334 = node-c288() -> ()  [unwired: 1 in, 1 out]
  }
  n1335 = node-c288() -> (w109:T25)  [unwired: 4 out]
  n1336 = timed-loop "Mouse control: trap position (AOM deflection), set confocal spot from image" {
    tunnel: [w2056] -> w69
    tunnel: w59 -> [w2055]
    timing: w109 -> [_]
    timing-out: [_] -> w108
    stop <- w2056 stop-if-true
    n1337 = node-c288() -> ()  [unwired: 2 out]
    n1338 = event shown="[0] \"Pane\": Mouse Down" {
      selector: _ -> [_ _]
      dyn-events: _ -> [_ _]
      timeout: _ -> [_ _]
      tunnel: w2055 -> [w2059 _]
      event Mouse Down {
        n1339 = event-data() -> ("Time"=w2061:u32, "Coords"=w2060:T8, "Button"=w2062:u16)  [unwired: 6 out]
        n1340 = case shown="3" w2062 {
          tunnel: w2061 -> [_ _ w2165]
          tunnel: w2060 -> [_ w2099 w2163]
          tunnel: w2059 -> [_ _ w2161]
          frame 0, Default {
          }
          frame 1 {
            n1341 = property on="APD 2" class="ImageControl"() -> ("Displayed Image Position"=w2069:cluster{"Left":i32, "Top":i32})  [unwired: 2 in, 2 out]
            n1342 = property on="APD 1" class="ImageControl"() -> ("Displayed Image Position"=w2098:cluster{"Left":i32, "Top":i32})  [unwired: 2 in, 2 out]
            n1343 = property on="Detection Laser X" class="ImageControl"() -> ("Displayed Image Position"=w2095:cluster{"Left":i32, "Top":i32})  [unwired: 2 in, 2 out]
            n1344 = property on="Detection Laser Y" class="ImageControl"() -> ("Displayed Image Position"=w2094:cluster{"Left":i32, "Top":i32})  [unwired: 2 in, 2 out]
            n1345 = property on="APD 2" class="ImageControl"() -> ("Displayed Image Size"=w2068:cluster{"Width":u32, "Height":u32})  [unwired: 2 in, 2 out]
            n1346 = property on="APD 1" class="ImageControl"() -> ("Displayed Image Size"=w2096:cluster{"Width":u32, "Height":u32})  [unwired: 2 in, 2 out]
            n1347 = property on="Detection Laser X" class="ImageControl"() -> ("Displayed Image Size"=w2097:cluster{"Width":u32, "Height":u32})  [unwired: 2 in, 2 out]
            n1348 = property on="Detection Laser Y" class="ImageControl"() -> ("Displayed Image Size"=w2093:cluster{"Width":u32, "Height":u32})  [unwired: 2 in, 2 out]
            n1349 = Unbundle By Name(w2068) -> ("Width"=w2065:u32, "Height"=w2064:u32)
            n1350 = Unbundle By Name(w2069) -> ("Left"=w2067:i32, "Top"=w2066:i32)
            n1351 = Unbundle By Name(w2096) -> ("Width"=w2090:u32, "Height"=w2089:u32)
            n1352 = Unbundle By Name(w2097) -> ("Width"=w2086:u32, "Height"=w2085:u32)
            n1353 = Unbundle By Name(w2093) -> ("Width"=w2082:u32, "Height"=w2081:u32)
            n1354 = Unbundle By Name(w2098) -> ("Left"=w2092:i32, "Top"=w2091:i32)
            n1355 = Unbundle By Name(w2095) -> ("Left"=w2088:i32, "Top"=w2087:i32)
            n1356 = Unbundle By Name(w2094) -> ("Left"=w2084:i32, "Top"=w2083:i32)
            n1357 = Bundle("Left"=w2067, "Top"=w2066, "Width"=w2065, "Height"=w2064) -> (w2063:T34)  [unwired: 1 in]
            n1358 = Bundle("Left"=w2092, "Top"=w2091, "Width"=w2090, "Height"=w2089) -> (w2080:T34)  [unwired: 1 in]
            n1359 = Bundle("Left"=w2088, "Top"=w2087, "Width"=w2086, "Height"=w2085) -> (w2079:T34)  [unwired: 1 in]
            n1360 = Bundle("Left"=w2084, "Top"=w2083, "Width"=w2082, "Height"=w2081) -> (w2078:T34)  [unwired: 1 in]
            n1361 = Build Cluster Array(w2063, w2080, w2079, w2078) -> (w2077:T35)
            n1362 = for {
              tunnel: w2099 -> [w2110]
              tunnel: w2077 -> [w2111] mode=indexing
              shift-right: [w2108] -> w2075
              shift-left: TRUE -> [w2109]
              shift-right: [w2107] -> w2073
              shift-left: _ -> [w2103]
              shift-right: [w2106] -> w2072
              shift-left: _ -> [w2102]
              shift-right: [w2105] -> w2071
              shift-left: _ -> [w2101]
              shift-right: [w2104] -> w2070
              shift-left: _ -> [w2100]
              n1363 = case shown="True" w2109 {
                selector: w2109 -> [w2116 _]
                tunnel: w2111 -> [_ w2125]
                tunnel: w2110 -> [_ w2123]
                tunnel: [w2116 w2121] -> w2108
                tunnel: [w2115 w2120] -> w2107
                tunnel: [w2114 w2119] -> w2106
                tunnel: [w2113 w2118] -> w2105
                tunnel: [w2112 w2117] -> w2104
                tunnel: w2103 -> [w2115 _]
                tunnel: w2102 -> [w2114 _]
                tunnel: w2101 -> [w2113 _]
                tunnel: w2100 -> [w2112 _]
                frame False {
                }
                frame True {
                  n1364 = Unbundle(w2125) -> (w2124:T34)
                  n1365 = call "isclickinwindow.vi"("Image Param"=w2124, "Point32"=w2123) -> ("Y px"=w2117:i32, "Height"=w2118:i32, "X px"=w2119:i32, "Width"=w2120:i32, "In image?"=w2122:bool)  [unwired: 1 in]
                  n1366 = Not(x=w2122) -> (.not. x?=w2121:bool)
                }
              }
            }
            n1367 = Not(x=w2075) -> (.not. x?=w2074:bool)
            n1368 = case shown="True" w2074 {
              tunnel: w2072 -> [_ w2138]
              tunnel: w2070 -> [_ w2137]
